vi "Read GObject selectors.vi"(8 "Error in":errorcluster, 11 "Generic In":refnum<vi>) -> (0 "Error out":errorcluster, 3 "Selectors":string[](array[string]))   [LabVIEW 2019, in "LSS.lvlib"]
doc: "Read the selectors out of the Front Panel object reference input. \n\n<b>Inputs:</b>\n<b>Generic In</b> - Front Panel Object from which to read the selelctors.\n<b>Error In</b> - Standard Error In terminal.\n\n<b>Outputs:</b>\n<b>Selectors</b> - List of selectors that apply to the Object passed as an input.\n<b>Error Out</b> - Standard Error out terminal."
uses:
  LSS.lvlib
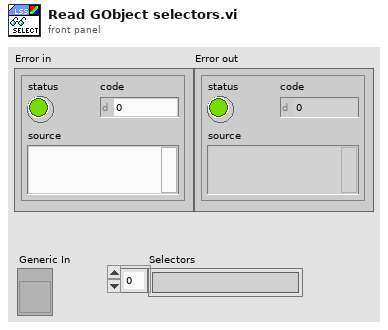
[diagram p1: front panel]
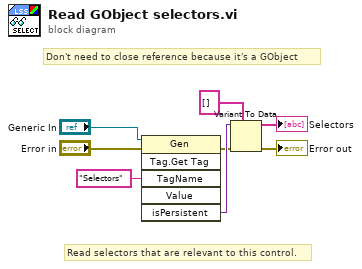
[diagram p0: block diagram]
diagram:
  # "Read selectors that are relevant to this control."
  # "Don't need to close reference because it's a GObject"
  n1 = invoke class="Gen" method="Tag.Get Tag"(reference="Generic In", error in="Error in", "TagName"="Selectors" ("Tag Name")) -> (error out=w2:errorcluster, "isPersistent"=w4:variant)  [unwired: 3 in, 4 out]
  n2 = Variant To Data(error in=w2, type=string[] [], Variant=w4) -> (data=→"Selectors":string[], error out=→"Error out":errorcluster)
